vi "Test Data is Sent to Listener.vi"(8 "error in (no error)":errorcluster, 11 "Test Case In":refnum<class "Debug Message Receiver Test.lvclass">) -> (0 "error out":errorcluster, 3 "Test Case Out":refnum<class "Debug Message Receiver Test.lvclass">)   [LabVIEW 2020, in "Debug Message Receiver Test.lvclass"]
uses:
  Debug Message Receiver Test.lvclass
  Debug Message Receiver Test.lvclass/Debug Message Receiver Test.ctl
  01074fa8-ee8a-411d-bc8b-fc92c4f90959.vi
  source/Process/Debug Process.lvclass
  source/Debug Message Receiver/Debug Message Receiver.lvclass
  C:/Users/anton/Documents/GitHub/triarc-debugger/source/Process/Debug Process.lvclass
  C:/Users/anton/Documents/GitHub/triarc-debugger/source/Debug Message Receiver/Debug Message Receiver.lvclass
  source/Mock Data Listener/Mock Data Listener.lvclass
  C:/Users/anton/Documents/GitHub/triarc-debugger/source/Mock Data Listener/Mock Data Listener.lvclass
  C:/Users/anton/Documents/GitHub/triarc-debugger/source/Debug Data Event/Debug Data Listener.lvclass
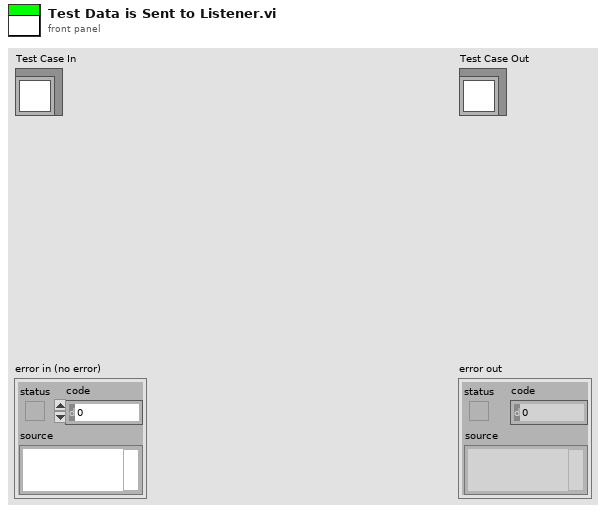
[diagram p1: front panel]
types:
  T1 = cluster{"Action":string, "Call Chain":string, "Process":string, "Message":string, "Message Data":variant, "Time":u32}
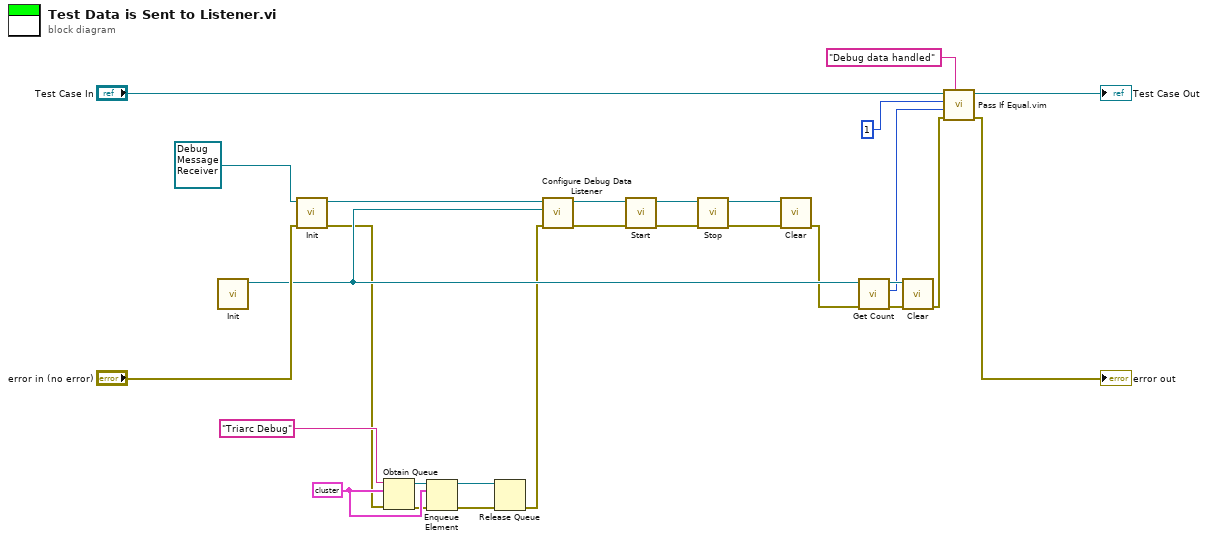
[diagram p0: block diagram]
diagram:
  w11 = T1 {"Action"="", "Call Chain"="", "Process"="", "Message"="", "Message Data"=variant, "Time"=0} ("output cluster")
  n1 = call "Init.vi"() -> ("Mock Data Listener Out"=w14:refnum<class "Mock Data Listener.lvclass">)  [unwired: 10 in, 1 out]
  n2 = call-dynamic "Init.vi"("error in (no error)"="error in (no error)", "Process In"=refnum<class "Debug Message Receiver.lvclass"> refnum ("Debug Message Receiver.lvclass")) -> ("error out"=w6:errorcluster, "Process Out"=w18:refnum<class "Debug Message Receiver.lvclass">)  [unwired: 8 in]
  n3 = Obtain Queue(name (unnamed)="Triarc Debug", element data type=w11, error in (no error)=w6) -> (queue out=w10:refnum<queue>, error out=w9:errorcluster)  [unwired: 2 in, 1 out]
  n4 = Enqueue Element(queue=w10, element=w11, error in (no error)=w9) -> (queue out=w8:refnum<queue>, error out=w7:errorcluster)  [unwired: 1 in, 1 out]
  n5 = Release Queue(queue=w8, error in (no error)=w7) -> (error out=w5:errorcluster)  [unwired: 1 in, 2 out]
  n6 = call "Configure Debug Data Listener.vi"("error in (no error)"=w5, "Debug Data Listener"=w14, "Debug Message Receiver In"=w18) -> ("error out"=w19:errorcluster, "Debug Message Receiver Out"=w20:refnum<class "Debug Message Receiver.lvclass">)  [unwired: 7 in]
  n7 = call "Start.vi"("error in (no error)"=w19, "Process In"=w20) -> ("error out"=w24:errorcluster, "Process Out"=w25:refnum<class "Debug Message Receiver.lvclass">)  [unwired: 7 in, 1 out]
  n8 = call "Stop.vi"("error in (no error)"=w24, "Process In"=w25) -> ("error out"=w22:errorcluster, "Process Out"=w23:refnum<class "Debug Message Receiver.lvclass">)  [unwired: 7 in, 1 out]
  n9 = call-dynamic "Clear.vi"("error in (no error)"=w22, "Process In"=w23) -> ("error out"=w13:errorcluster)  [unwired: 9 in]
  n10 = call "Get Count.vi"("error in (no error)"=w13, "Mock Data Listener In"=w14) -> ("error out"=w16:errorcluster, "Count"=w4:i32, "Mock Data Listener Out"=w15:refnum<class "Mock Data Listener.lvclass">)  [unwired: 7 in]
  n11 = call "Clear.vi"("error in (no error)"=w16, "Mock Data Listener in"=w15) -> ("error out"=w2:errorcluster)  [unwired: 9 in]
  n12 = call "Pass If Equal.vim"("Description"="Debug data handled", "error in (no error)"=w2, "Actual"=w4, "Expected"=1 ("Count"), "LUnit Test Case In"="Test Case In") -> ("error out"=→"error out":errorcluster, "LUnit Test Case Out"=→"Test Case Out":refnum<class "Debug Message Receiver Test.lvclass">)  [unwired: 5 in]
